vi "Get and save image.vi"(8 "error in (no error)":errorcluster, 10 "Camera Mod ID":i32, 11 "Path":path) -> (0 "error out":errorcluster, 3 "Image out":T1)   [LabVIEW 2020]
uses:
  Camera/Libraries/Camera/Camera.lvlib
  <vilib>/vision/Image Controls.llb/IMAQ Image.ctl
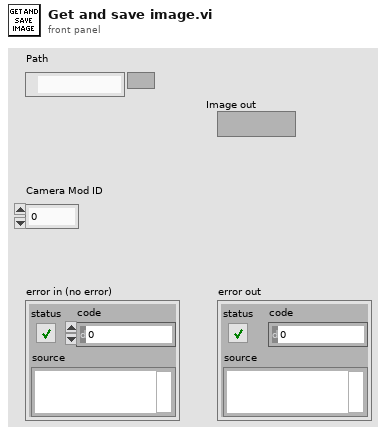
[diagram p1: front panel]
types:
  T1 = typedef "IMAQ Image.ctl" = refnum<image>
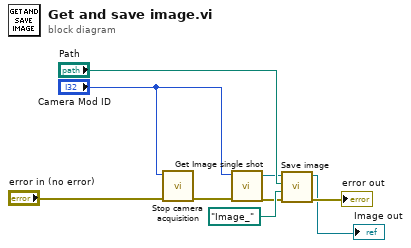
[diagram p0: block diagram]
diagram:
  n1 = call "Stop camera acquisition.vi"("error in"="error in (no error)", "Module ID"="Camera Mod ID") -> ("error out"=w8:errorcluster)  [unwired: 9 in]
  n2 = call "Get Image single shot.vi"("error in"=w8, "Module ID"="Camera Mod ID") -> ("error out"=w2:errorcluster, "Image"=w3:T1)  [unwired: 7 in, 1 out]
  n3 = call "Save image.vi"("error in (no error)"=w2, "Base name"=path "Image_", "Path"="Path", "Image in"=w3) -> ("error out"=→"error out":errorcluster, "Image out"=→"Image out":T1)  [unwired: 6 in]
